vi "Main.vi"() -> ()   [LabVIEW 2018, in "TestStand_Control.lvlib"]
doc: "This template is based off of the Queued Message Handler design pattern and the Queued Message Handler project template that ships with LabVIEW.\n\nThe main difference is that the queue is private to this module and communication between modules is performed via Broadcast and Request events.\n\nRequest events are wrapped in public API methods and are handled in the Event Handling Loop (EHL) of this VI. Any module can register for Broadcast events sent by this module. The EHL generates messages based on user interface actions.\n\nThe Message Handling Loop (MHL) processes messages generated by the EHL, or by other messages. The messages are string values, so new messages can be added easily to the Message Cases case structure in the MHL. Each message cluster can also provide an optional value for Message Data, which is a variant that can be converted to whatever message-specific data is required.\n_____\nBased on Delacor QMH Project Template 4.2.1.64."
uses:
  TestStand_Control.lvlib
  <vilib>/Delacor/Delacor QMH/Libraries/Module Admin_class/Delacor_lib_QMH_Module Admin.lvclass
  Module Data--cluster.ctl
  Module_Controls/TestStand UI Data.ctl
  Stop Argument--cluster.ctl
  <vilib>/Delacor/Delacor QMH/Libraries/Message Queue_class/Delacor_lib_QMH_Message Queue.lvclass/Delacor_lib_QMH_Message Queue.ctl
  <vilib>/Delacor/Delacor QMH/Libraries/Module Admin_class/Delacor_lib_QMH_Module Admin.lvclass/Delacor_lib_QMH_Module Admin.ctl
  User_Selected_TestCase Argument--cluster.ctl
  Start_Execution Argument--cluster.ctl
  <vilib>/Utility/miscctls.llb/LVPointTypeDef.ctl
  <vilib>/Delacor/Delacor QMH/Libraries/Message Queue_class/Delacor_lib_QMH_Enqueue Message (Single).vi
  <vilib>/Delacor/Delacor QMH/Libraries/Module Admin_class/Delacor_lib_QMH_Get External Launch.vi
  <vilib>/Utility/error.llb/Error Cluster From Error Code.vi
  <vilib>/ErrorRing/Error Ring.xnode
  <vilib>/Delacor/Delacor QMH/Libraries/Message Queue_class/Delacor_lib_QMH_Message Queue.lvclass
panel:
  in  "Subpanel Ref":refnum<vi>
  in  "TestStand UI SequenceView Control":refnum<k7>(container)
  in  "Path":path
  in  "Entry Point 1 Button":refnum<k7>(container)
  in  "Start":bool
  in  "Break":refnum<k7>(container)
  in  "Terminate":refnum<k7>(container)
  in  "Test_Case":string
  in  "SequenceView Control":refnum<k7>(container)
  in  "ExecutionView Manager":refnum<k7>(container)
  in  "SequenceFileView Manager":refnum<k7>(container)
  in  "Application Manager":refnum<k7>(container)
  out "error out":errorcluster
  in  "Module Admin":refnum<class "Delacor_lib_QMH_Module Admin.lvclass">
  out "Status":string
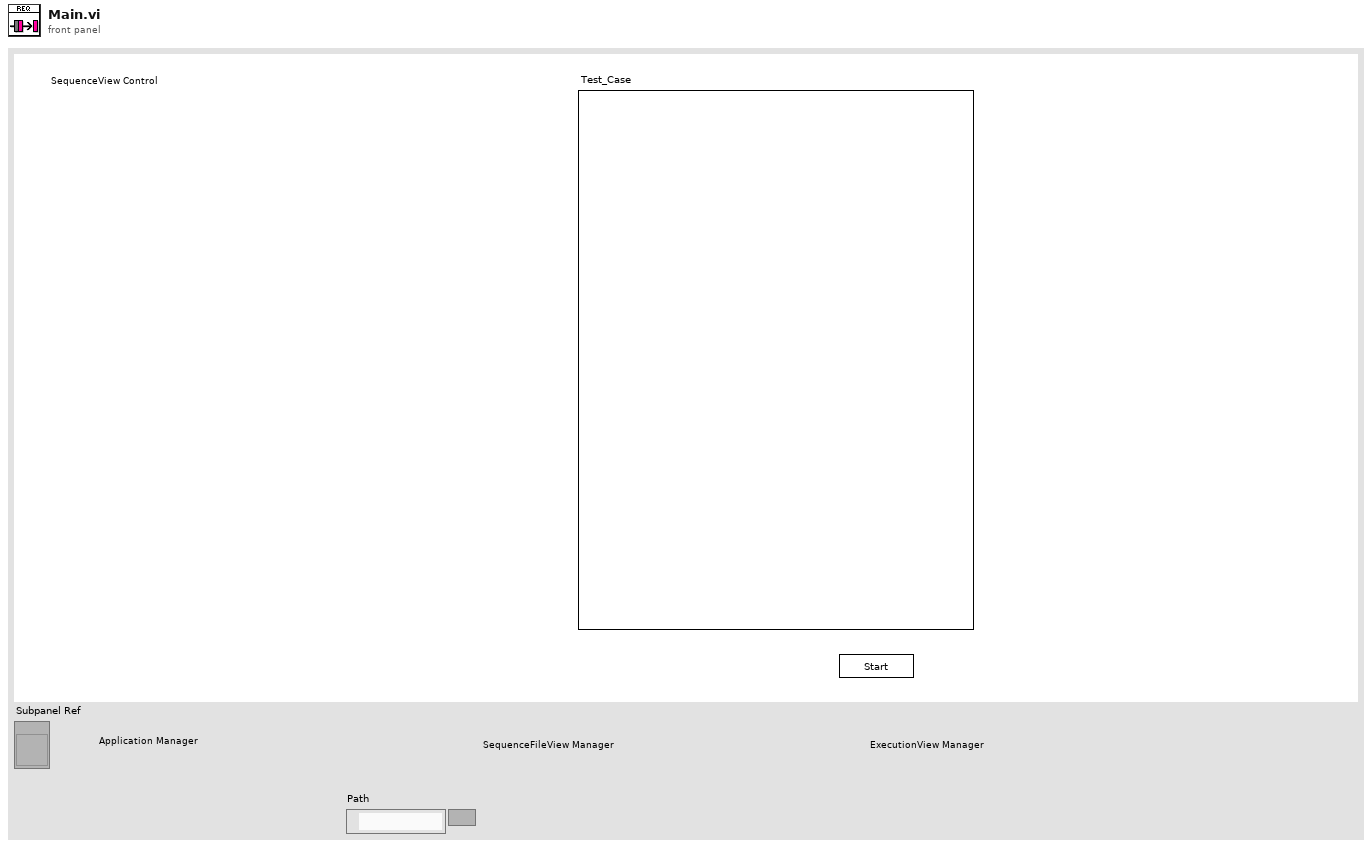
[diagram p1: front panel]
types:
  T1 = typedef "TestStand_Control.lvlib/Module Data--cluster.ctl" = cluster{"Status":string, "TestStand UI Data":T2, "Test_ID":string[], "Test_ID User":string[], "Test_Case":string[], "Subpanel Ref":refnum<vi>, "Working_Directory":path}
  T2 = typedef "TestStand_Control.lvlib/TestStand UI Data.ctl" = cluster{"Other References":cluster{"Event Callback":refnum<k27>, "Quit Application Event":refnum<user-event>, "Event Reg Refnum":refnum<event-registration>, "Top level VI":refnum<vi>, "TestStand Engine":refnum<k7>}, "Manager Controls":cluster{"Application Manager":refnum<k7>, "SequenceFileView Manager":refnum<k7>, "ExecutionView Manager":refnum<k7>}, "Visible Controls":cluster{"Terminate/Restart Button":refnum<k7>, "Break/Resume Button":refnum<k7>, "Close Executions Button":refnum<k7>, "Report Viewer":refnum<k7>, "Execution View":refnum<k7>, "Executions ComboBox":refnum<k7>, "Run Selected Sequence Button":refnum<k7>, "Entry Point 2 Button":refnum<k7>, "Entry Point 1 Button":refnum<k7>, "Close Sequence File Button":refnum<k7>, "Open Sequence File Button":refnum<k7>, "Sequences ComboBox":refnum<k7>, "Sequence Files ComboBox":refnum<k7>, "Terminate All Button":refnum<k7>, "Exit Button":refnum<k7>, "Login/Logout Button":refnum<k7>}}
  T3 = typedef "TestStand_Control.lvlib/Request Events--cluster.ctl" = cluster{"Stop Module":refnum<user-event>, "Show Panel":refnum<user-event>, "Hide Panel":refnum<user-event>, "Get Module Execution Status":refnum<user-event>, "Show Diagram":refnum<user-event>, "User_Selected_TestCase":refnum<user-event>, "Start_Execution":refnum<user-event>}
  T4 = enum32{"invalid lock state", "Not Locked", "Locked (No Password)", "Password-protected"}
  T5 = typedef "TestStand_Control.lvlib/Stop Argument--cluster.ctl" = cluster{"Origin":string, "Exit via Stop Module Req?":bool, "Wait for Module to stop?":bool}
  T6 = enum8{"Enabled", "Disabled", "Disabled and Grayed Out"}
  T7 = typedef "TestStand_Control.lvlib/User_Selected_TestCase Argument--cluster.ctl" = cluster{"Test_Case_ID":string[]}
  T8 = typedef "TestStand_Control.lvlib/Start_Execution Argument--cluster.ctl" = cluster{"Start":bool}
  T9 = typedef "LVPointTypeDef.ctl" = cluster{"Horizontal":i16, "Vertical":i16}
  T10 = enum32{"Invalid", "Standard", "Closed", "Hidden", "Minimized", "Maximized"}
  T11 = cluster{"test_id":string, "status":string, "report":string, "last":bool}
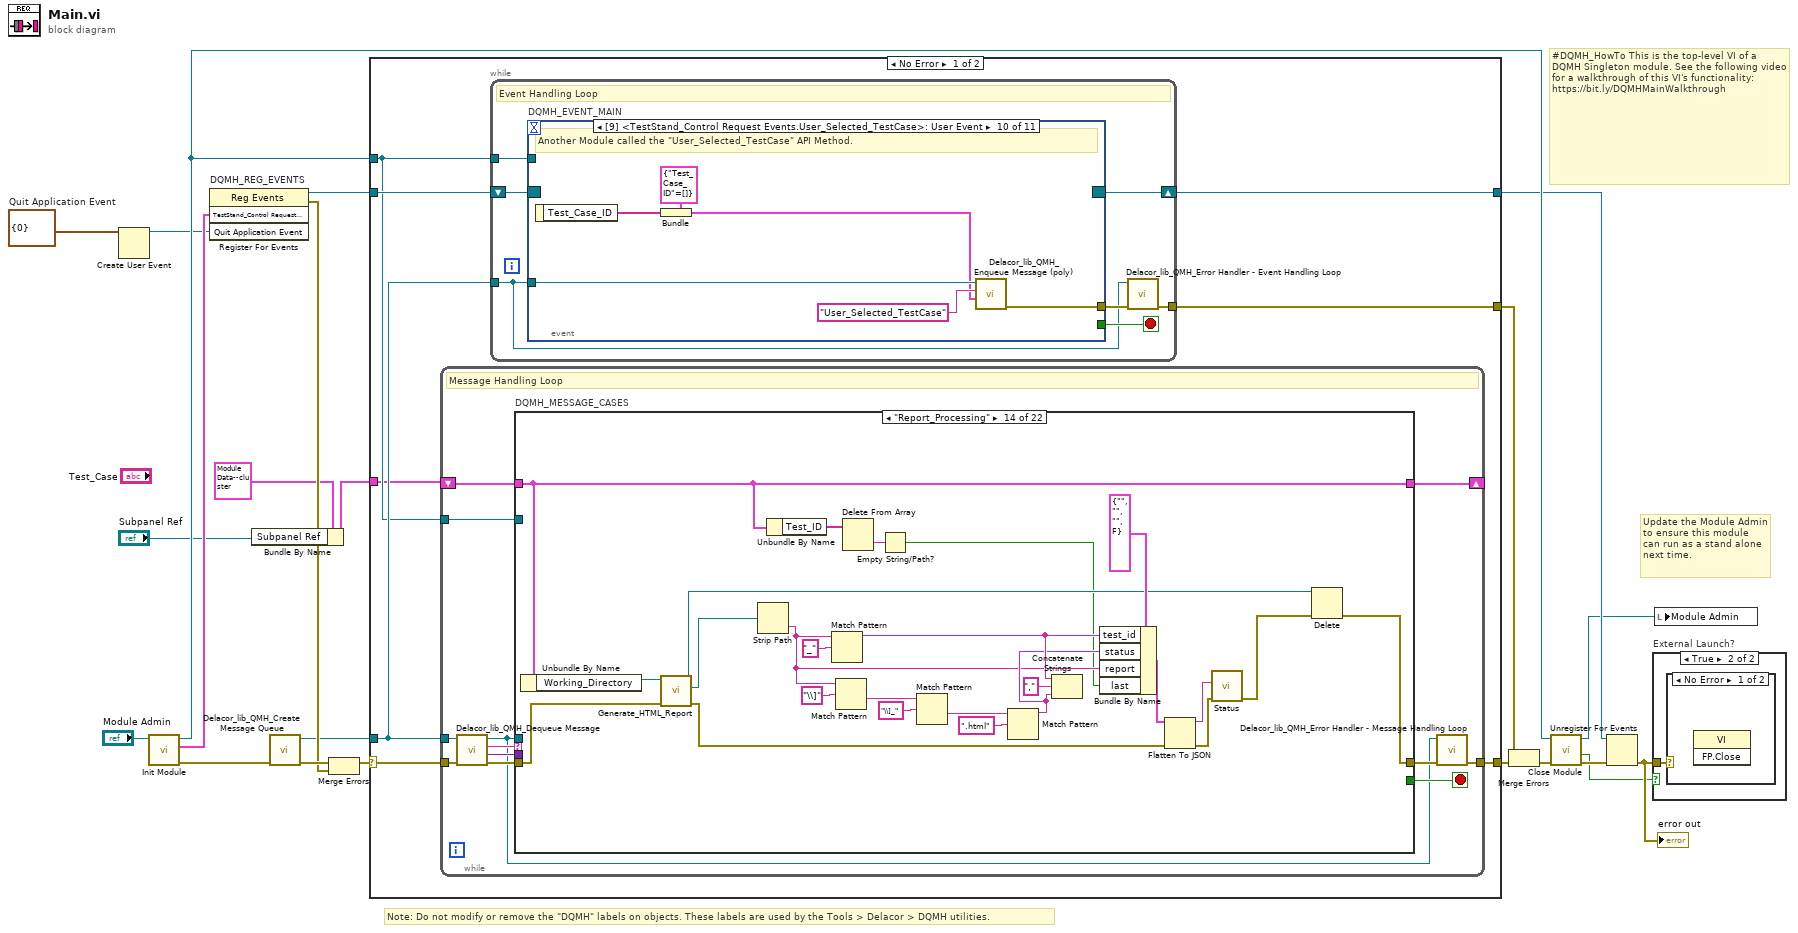
[diagram p0: block diagram]
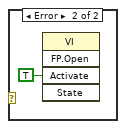
[diagram p3: hidden frame]
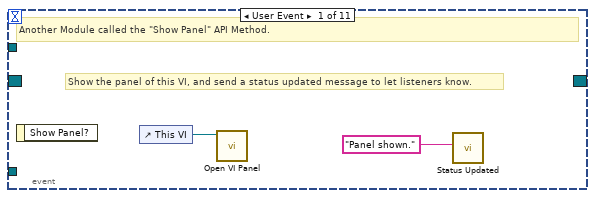
[diagram p4: hidden frame]
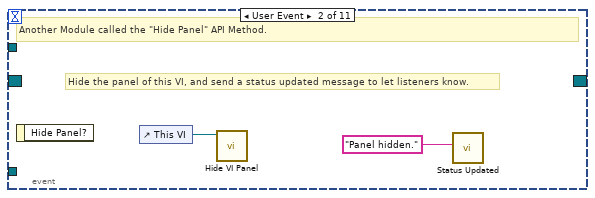
[diagram p5: hidden frame]
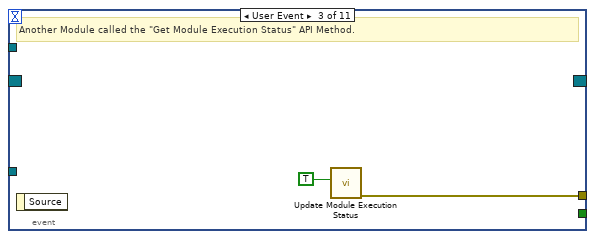
[diagram p6: hidden frame]
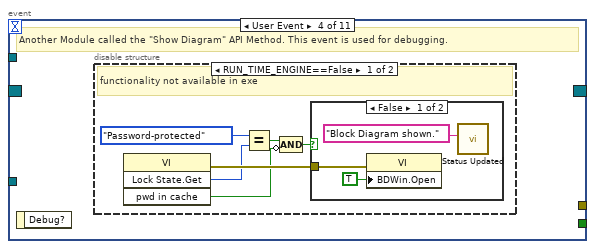
[diagram p7: hidden frame]
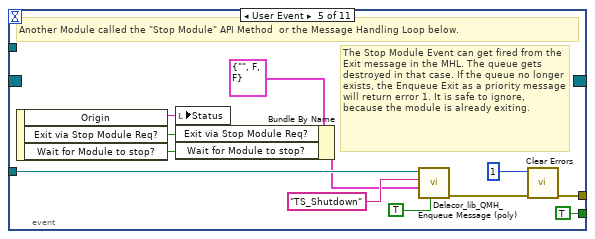
[diagram p10: hidden frame]
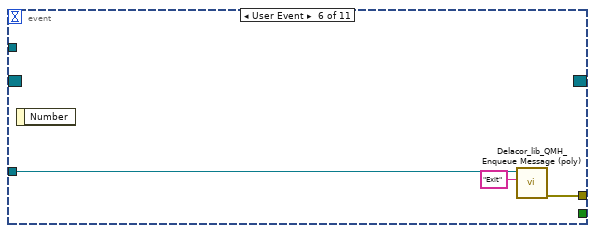
[diagram p11: hidden frame]
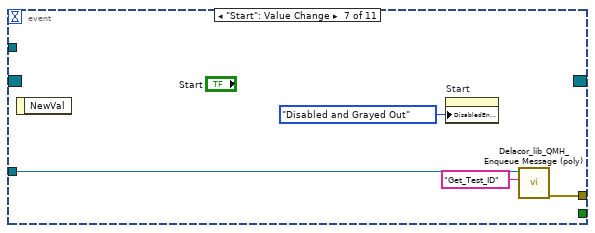
[diagram p12: hidden frame]
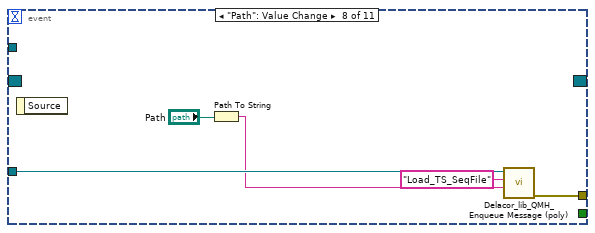
[diagram p13: hidden frame]
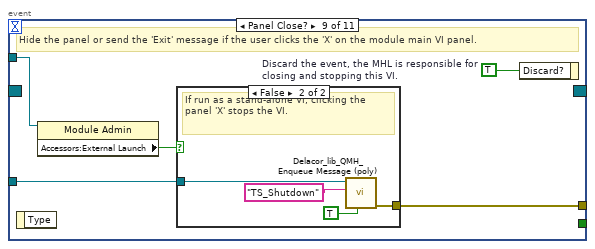
[diagram p14: hidden frame]
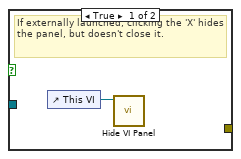
[diagram p15: hidden frame]
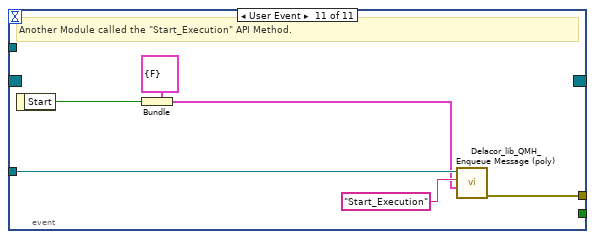
[diagram p16: hidden frame]
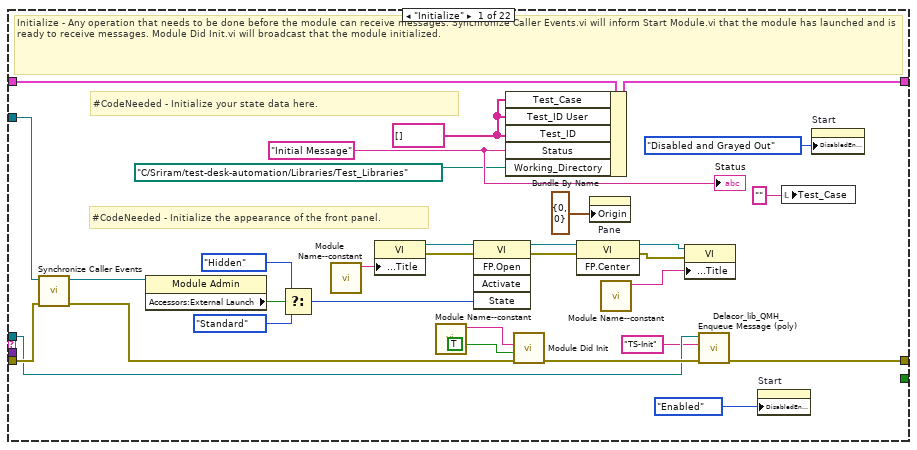
[diagram p17: hidden frame]
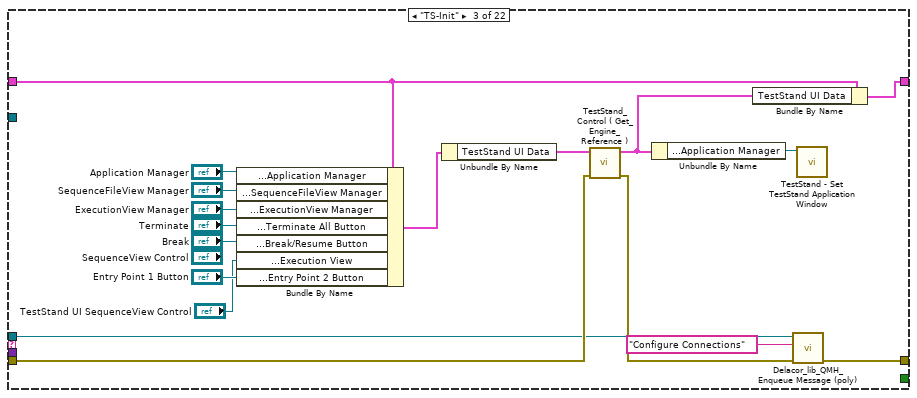
[diagram p19: hidden frame]
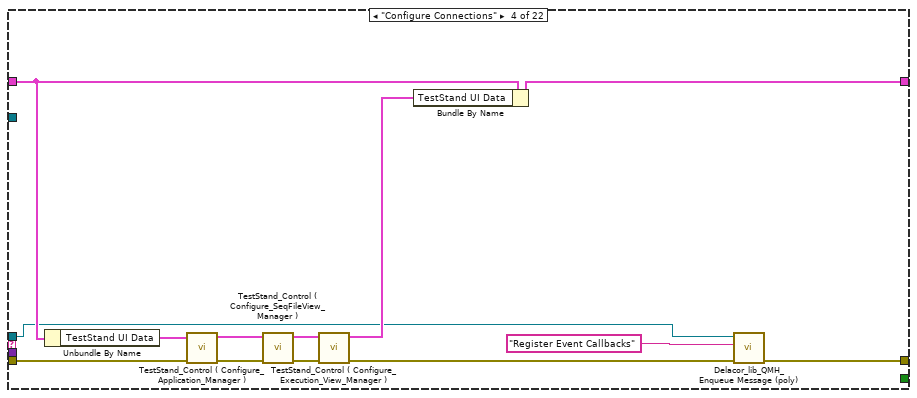
[diagram p20: hidden frame]
diagram:
  w5 = cluster{"Number":i32} {"Number"=0}  # Quit Application Event
  # "#DQMH_HowTo This is the top-level VI of a DQMH Singleton module. See the following video for a walkthrough of this VI's functionality: https://bit.ly/DQMHMainWalkthrough"
  # "Note: Do not modify or remove the \"DQMH\" labels on objects. These labels are used by the Tools > Delacor > DQMH utilities."
  # "Update the Module Admin to ensure this module can run as a stand alone next time."
  n1 = Create User Event(user event datatype=w5) -> (user event=w4:refnum<user-event>)  [unwired: 1 in, 1 out]
  n2 = call "Init Module.vi"("Singleton Module Admin in"="Module Admin") -> ("error out"=w21:errorcluster, "TestStand_Control Request Events"=w10:T3, "Singleton Module Admin out"=w13:refnum<class "Delacor_lib_QMH_Module Admin.lvclass">)  [unwired: 8 in]
  n3 = register-events "DQMH_REG_EVENTS"(w10, w4) -> (reference out=w11:refnum<event-registration>, error out=w14:errorcluster)  [unwired: 2 in]
  n4 = Bundle By Name(cluster=T1 {"Status"="", "TestStand UI Data"={"Other References"={"Event Callback"=refnum, "Quit Application Event"=refnum, "Event Reg Refnum"=refnum, "Top level VI"=refnum, "TestStand Engine"=refnum}, "Manager Controls"={"Application Manager"=refnum, "SequenceFileView Manager"=refnum, "ExecutionView Manager"=refnum}, "Visible Controls"={"Terminate/Restart Button"=refnum, "Break/Resume Button"=refnum, "Close Executions Button"=refnum, "Report Viewer"=refnum, "Execution View"=refnum, "Executions ComboBox"=refnum, "Run Selected Sequence Button"=refnum, "Entry Point 2 Button"=refnum, "Entry Point 1 Button"=refnum, "Close Sequence File Button"=refnum, "Open Sequence File Button"=refnum, "Sequences ComboBox"=refnum, "Sequence Files ComboBox"=refnum, "Terminate All Button"=refnum, "Exit Button"=refnum, "Login/Logout Button"=refnum}}, "Test_ID"=[], "Test_ID User"=[], "Test_Case"=[], "Subpanel Ref"=refnum, "Working_Directory"=path ""} ("Data Cluster"), "Subpanel Ref"="Subpanel Ref") -> (w2:T1)
  n5 = call <vilib>:"Delacor_lib_QMH_Create Message Queue.vi"("error in (no error)"=w21) -> ("error out"=w16:errorcluster, "Message Queue"=w9:refnum<class "Delacor_lib_QMH_Message Queue.lvclass">)  [unwired: 9 in]
  n6 = Merge Errors(w16, w14) -> (w15:errorcluster)
  n7 = case shown="No Error" w15 {
    selector: w15 -> [w28 w423]
    tunnel: [w30 w423] -> w22
    tunnel: [w27 w420] -> w12
    tunnel: w11 -> [w26 w420]
    tunnel: w9 -> [w25 _]
    tunnel: [w29 _] -> w19
    tunnel: w13 -> [w24 w416]
    tunnel: w2 -> [w23 _]
    frame No Error {
      n8 = while {
        tunnel: w25 -> [w101]
        shift-right: [w105] -> _
        shift-left: w23 -> [w106]
        tunnel: w28 -> [w109]
        tunnel: [w107] -> w30
        tunnel: w24 -> [w99]
        stop <- w104 stop-if-true
        # "Message Handling Loop"
        n9 = call-dynamic "Delacor_lib_QMH_Dequeue Message.vi"("error in (no error)"=w109, "Message Queue in"=w101) -> ("error out"=w108:errorcluster, "Message Data"=w102:variant, "Message"=w103:string, "Message Queue out"=w100:refnum<class "Delacor_lib_QMH_Message Queue.lvclass">)  [unwired: 6 in]
        n10 = case "DQMH_MESSAGE_CASES" shown="\"Report_Processing\"" w103 {
          selector: w103 -> [_ _ _ _ _ _ _ _ _ _ _ _ _ _ _ _ _ _ _ _ _ w403]
          tunnel: w100 -> [w121 _ w150 w162 w179 _ w202 _ _ _ _ w262 w272 _ w307 w322 w341 _ _ w369 w396 _]
          tunnel: w108 -> [w139 w143 w153 w174 w180 w190 w204 w222 w246 w249 w258 w264 w273 w301 w305 w340 w349 w364 w366 w376 w401 w405]
          tunnel: [w122 w143 w152 w164 w181 w190 w203 w223 w239 w247 w257 w263 w266 w300 w310 w318 w343 w363 w366 w372 w399 w406] -> w110
          tunnel: w106 -> [w129 w142 w147 w172 w189 w193 w205 w227 w238 w250 w252 w259 w276 w280 w313 w334 w348 w362 w365 w371 w384 w404]
          tunnel: [w112 w142 w146 w167 w188 w193 w200 w226 w238 w250 w252 w259 w276 w280 w313 w330 w348 w362 w365 w371 w384 w404] -> w105
          tunnel: [_ _ _ _ _ _ _ _ _ _ _ _ _ _ _ _ _ _ _ _ w395 _] -> w104
          tunnel: w102 -> [_ _ _ _ _ _ _ _ w243 _ w255 _ _ _ _ w339 w347 _ _ w370 w394 _]
          tunnel: w99 -> [w130 _ _ _ _ _ _ _ _ _ _ _ _ _ _ _ _ _ _ w368 w389 _]
          frame "Initialize" {
            w116 = string[] [] ("Test_ID")
            w124 = "Initial Message" ("Initial Message")
            # "#CodeNeeded - Initialize the appearance of the front panel."
            # "#CodeNeeded - Initialize your state data here."
            # "Initialize - Any operation that needs to be done before the module can receive messages. Synchronize Caller Events.vi will inform Start Module.vi that the module has launched and is ready to receive messages. Module Did Init.vi will broadcast that the module initialized."
            n11 = call "Synchronize Caller Events.vi"("error in (no error)"=w139, "Singleton Module Admin in"=w130) -> ("error out"=w138:errorcluster, "Singleton Module Admin out"=w126:refnum<class "Delacor_lib_QMH_Module Admin.lvclass">)  [unwired: 8 in]
            n12 = property class="Module Admin"(reference=w126) -> ("Accessors:External Launch"=w134:bool)  [unwired: 1 in, 2 out]
            n13 = Select(t=T10."Hidden" ("State"), s=w134, f=T10."Standard" ("State")) -> (s? t:f=w131:T10)
            n14 = call "Module Name--constant.vi"() -> ("Module Name"=w137:string)  [unwired: 11 in]
            n15 = property class="VI"("Front Panel.Title"=w137) -> (reference out=w136:refnum<vi>, error out=w141:errorcluster)  [unwired: 2 in]
            n16 = call "Module Name--constant.vi"() -> ("Module Name"=w127:string)  [unwired: 11 in]
            n17 = invoke class="VI" method="FP.Open"(reference=w136, error in=w141, "State"=w131) -> (reference out=w135:refnum<vi>, error out=w140:errorcluster)  [unwired: 2 in, 3 out]
            n18 = Bundle By Name(cluster=w129, "Test_Case"=w116, "Test_ID User"=w116, "Test_ID"=w116, "Status"=w124, "Working_Directory"=path "C:/Sriram/test-desk-automation/Libraries/Test_Libraries") -> (w112:T1)
            n19 = call "Module Did Init.vi"("error in (no error)"=w138, "Initialized?"=TRUE, "Origin"=w127) -> ("error out"=w123:errorcluster)  [unwired: 8 in]
            n20 = invoke class="VI" method="FP.Center"(reference=w135, error in=w140) -> (reference out=w114:refnum<vi>, error out=w115:errorcluster)  [unwired: 1 in, 1 out]
            n21 = property on="Pane" class="Pane"("Origin"=T9 {"Horizontal"=0, "Vertical"=0}) -> ()  [unwired: 2 in, 2 out]
            n22 = call "Module Name--constant.vi"() -> ("Module Name"=w113:string)  [unwired: 11 in]
            n23 = property class="VI"(reference=w114, error in=w115, "Front Panel.Title"=w113) -> ()  [unwired: 2 out]
            n24 = call-poly <vilib>:"Delacor_lib_QMH_Enqueue Message (poly).vi"("error in (no error)"=w123, "Message"="TS-Init", "Message Queue in"=w121) -> ("error out"=w122:errorcluster)  [unwired: 7 in, 1 out]
            n25 = property on="Start" class="Bool"("DisabledEnum"=T6."Enabled" ("Disabled")) -> ()  [unwired: 2 in, 2 out]
            n26 = local write "Test_Case"("" ("Test_Case")) -> ()
            n27 = property on="Start" class="Bool"("DisabledEnum"=T6."Disabled and Grayed Out" ("Disabled")) -> ()  [unwired: 2 in, 2 out]
            "Status" <- w124
          }
          frame "--- Module Specific ---" {
            # "Separator -- The following cases handle messages specific to this Module."
          }
          frame "TS-Init" {
            n28 = Bundle By Name(cluster=w147, "TestStand UI Data.Manager Controls.Application Manager"="Application Manager", "TestStand UI Data.Manager Controls.SequenceFileView Manager"="SequenceFileView Manager", "TestStand UI Data.Manager Controls.ExecutionView Manager"="ExecutionView Manager", "TestStand UI Data.Visible Controls.Terminate All Button"="Terminate", "TestStand UI Data.Visible Controls.Break/Resume Button"="Break", "TestStand UI Data.Visible Controls.Execution View"="TestStand UI SequenceView Control", "TestStand UI Data.Visible Controls.Entry Point 2 Button"="Entry Point 1 Button") -> (w155:T1)
            n29 = Unbundle By Name(w155) -> ("TestStand UI Data"=w154:T2)
            n30 = call "TestStand_Control ( Get_Engine_Reference ).vi"("error IO"=w153, "TestStand UI Data"=w154) -> ("error IO 2"=w151:errorcluster, "TestStand UI Data 2"=w145:T2)  [unwired: 8 in]
            n31 = Unbundle By Name(w145) -> ("Manager Controls.Application Manager"=w161:refnum<k7>)
            n32 = Bundle By Name(cluster=w147, "TestStand UI Data"=w145) -> (w146:T1)
            n33 = call-poly <vilib>:"Delacor_lib_QMH_Enqueue Message (poly).vi"("error in (no error)"=w151, "Message"="Configure Connections", "Message Queue in"=w150) -> ("error out"=w152:errorcluster)  [unwired: 7 in, 1 out]
            n34 = call <vilib>:"TestStand - Set TestStand Application Window.vi"("Application Manager"=w161) -> ()  [unwired: 2 in, 9 out]
          }
          frame "Configure Connections" {
            n35 = Unbundle By Name(w172) -> ("TestStand UI Data"=w171:T2)
            n36 = call "TestStand_Control ( Configure_Application_Manager ).vi"("error IO"=w174, "TestStand UI Data"=w171) -> ("error IO 2"=w173:errorcluster, "TestStand UI Data 2"=w169:T2)  [unwired: 8 in]
            n37 = call "TestStand_Control ( Configure_SeqFileView_Manager ).vi"("error IO"=w173, "TestStand UI Data"=w169) -> ("error IO"=w170:errorcluster, "TestStand UI Data 2"=w168:T2)  [unwired: 8 in]
            n38 = call "TestStand_Control ( Configure_Execution_View_Manager ).vi"("error IO 2"=w170, "TestStand UI Data"=w168) -> ("error IO"=w163:errorcluster, "TestStand UI Data 2"=w166:T2)  [unwired: 8 in]
            n39 = Bundle By Name(cluster=w172, "TestStand UI Data"=w166) -> (w167:T1)
            n40 = call-poly <vilib>:"Delacor_lib_QMH_Enqueue Message (poly).vi"("error in (no error)"=w163, "Message"="Register Event Callbacks", "Message Queue in"=w162) -> ("error out"=w164:errorcluster)  [unwired: 7 in, 1 out]
          }
          frame "Register Event Callbacks" {
            n41 = vi-ref "TestStand_Control ( Display_Sequence_Callback ).vi"() -> ("vi reference"=w185:refnum<vi>)
            n42 = vi-ref "TestStand_Control ( End_Execution ).vi"() -> ("vi reference"=w182:refnum<vi>)
            n43 = vi-ref "TestStand_Control ( Execution_View_Callback ).vi"() -> ("vi reference"=w184:refnum<vi>)
            n44 = vi-ref "TestStand_Control ( Start_Execution ).vi"() -> ("vi reference"=w183:refnum<vi>)
            n45 = vi-ref "TestStand_Control ( Exit_Callback ).vi"() -> ("vi reference"=w186:refnum<vi>)
            n46 = vi-ref "TestStand_Control ( Display_Execution ).vi"() -> ("vi reference"=w175:refnum<vi>)
            n47 = Unbundle By Name(w189) -> ("TestStand UI Data.Manager Controls.Application Manager"=w177:refnum<k7>, "TestStand UI Data"=w176:T2)
            n48 = node(w177, w185, w176, w177, w186, w176, w177, w184, w176, w177, w183, w179, w177, w182, w179, w177, w175, w176) -> (w187:refnum<k27>)  [unwired: 2 in, 1 out]
            n49 = call-poly <vilib>:"Delacor_lib_QMH_Enqueue Message (poly).vi"("error in (no error)"=w180, "Message"="Start Application", "Message Queue in"=w179) -> ("error out"=w181:errorcluster)  [unwired: 7 in, 1 out]
            n50 = Bundle By Name(cluster=w189, "TestStand UI Data.Other References.Event Callback"=w187) -> (w188:T1)
          }
          frame "Start Application" {
            n51 = Unbundle By Name(w193) -> ("TestStand UI Data.Manager Controls.Application Manager"=w194:refnum<k7>)
            n52 = invoke class="IApplicationMgr" method="Start"(reference=w194, error in=w190) -> (error out=w191:errorcluster)  [unwired: 1 in, 2 out]
            n53 = property on="Start" class="Bool"(error in=w191, "DisabledEnum"=T6."Enabled" ("Disabled")) -> ()  [unwired: 1 in, 2 out]
          }
          frame "Get_Test_ID" {
            n54 = Unbundle By Name(w205) -> ("Test_ID"=w201:string[], "Test_Case"=w196:string[])
            n55 = Delete From Array(array=w196) -> (deleted portion=w195:string)  [unwired: 2 in, 1 out]
            n56 = Delete From Array(array=w201) -> (deleted portion=w197:string, array with subset deleted=w199:string[])  [unwired: 2 in]
            n57 = Empty String/Path?(string/path=w197) -> (empty?=w198:bool)
            n58 = local write "Test_Case"(w195) -> ()
            n59 = case shown="False" w198 {
              tunnel: w204 -> [w217 w221]
              tunnel: [w212 w220] -> w203
              tunnel: w202 -> [w216 w219]
              tunnel: w197 -> [w214 _]
              frame False {
                n60 = call-poly <vilib>:"Delacor_lib_QMH_Enqueue Message (poly).vi"("error in (no error)"=w217, "Message Data"=w214, "Message"="Load_TS_SeqFile", "Message Queue in"=w216) -> ("error out"=w209:errorcluster, "Message Queue out"=w207:refnum<class "Delacor_lib_QMH_Message Queue.lvclass">)  [unwired: 6 in]
                n61 = call-poly <vilib>:"Delacor_lib_QMH_Enqueue Message (poly).vi"("error in (no error)"=w209, "Message Data"="TS_SetSeqView" ("Message"), "Message"="Switch_View", "Message Queue in"=w207) -> ("error out"=w208:errorcluster, "Message Queue out"=w206:refnum<class "Delacor_lib_QMH_Message Queue.lvclass">)  [unwired: 6 in]
                n62 = call-poly <vilib>:"Delacor_lib_QMH_Enqueue Message (poly).vi"("error in (no error)"=w208, "Message"="Trigger", "Message Queue in"=w206) -> ("error out"=w212:errorcluster)  [unwired: 7 in, 1 out]
              }
              frame True {
                n63 = call-poly <vilib>:"Delacor_lib_QMH_Enqueue Message (poly).vi"("error in (no error)"=w221, "Message"="Completed", "Message Queue in"=w219) -> ("error out"=w220:errorcluster)  [unwired: 7 in, 1 out]
              }
            }
            n64 = Bundle By Name(cluster=w205, "Test_ID"=w199) -> (w200:T1)
          }
          frame "Completed" {
            n65 = disable-structure shown="Disabled" {
              disable-tunnel: [w232 _] -> w223
              disable-tunnel: w222 -> [w231 _]
              frame Disabled {
                n66 = Flatten To JSON(anything=cluster{"status":string} {"status"="finished"}, error in (no error)=w231) -> (JSON string=w228:string, 11:w229:errorcluster)  [unwired: 1 in]
                n67 = call "Status.vi"("error in (no error)"=w229, "TS_Status"=w228) -> ("error out"=w232:errorcluster)  [unwired: 9 in]
              }
              frame Enabled {
              }
            }
            n68 = property on="Start" class="Bool"("DisabledEnum"=T6."Enabled" ("Disabled")) -> ()  [unwired: 2 in, 2 out]
            n69 = Bundle By Name(cluster=w227, "Test_ID"=string[] []) -> (w226:T1)
          }
          frame "Load_TS_SeqFile" {
            n70 = Variant To Data(error in=w246, type="", Variant=w243) -> (data=w241:string, error out=w244:errorcluster)
            n71 = Unbundle By Name(w238) -> ("Working_Directory"=w236:path)
            n72 = Concatenate Strings("TestBuilds\\" ("string"), w241, ".seq" ("string")) -> (w235:string)
            n73 = Build Path(base path=w236, name or relative path=w235) -> (appended path=w234:path)
            n74 = Unbundle By Name(w238) -> ("TestStand UI Data"=w245:T2)
            n75 = Path To String(path=w234) -> (string=w233:string)
            n76 = call "TestStand_Control ( Load_Seq_File ).vi"("error in (no error)"=w244, "sequenceFilePath"=w233, "TestStand UI Data"=w245) -> ("error out"=w239:errorcluster)  [unwired: 8 in]
          }
          frame "Trigger" {
            n77 = Unbundle By Name(w250) -> ("TestStand UI Data.Visible Controls.Entry Point 2 Button"=w248:refnum<k7>)
            n78 = invoke class="IButton" method="DoClick"(reference=w248, error in=w249) -> (error out=w247:errorcluster)  [unwired: 1 in, 2 out]
          }
          frame "Switch_View" {
            n79 = Variant To Data(error in=w258, type="", Variant=w255) -> (data=w253:string, error out=w256:errorcluster)
            n80 = Unbundle By Name(w252) -> ("TestStand UI Data"=w251:T2)
            n81 = call "TestStand_Control ( Switch_View ).vi"("error in"=w256, "View"=w253, "TestStand UI Data"=w251) -> ("error out"=w257:errorcluster)  [unwired: 8 in]
          }
          frame "TS_Execution_Start" {
            n82 = call-poly <vilib>:"Delacor_lib_QMH_Enqueue Message (poly).vi"("error in (no error)"=w264, "Message Data"="TS_SetExecView" ("Message"), "Message"="Switch_View", "Message Queue in"=w262) -> ("error out"=w263:errorcluster)  [unwired: 6 in, 1 out]
          }
          frame "TS_Execution_Stop" {
            n83 = call-poly <vilib>:"Delacor_lib_QMH_Enqueue Message (poly).vi"("error in (no error)"=w273, "Message Data"="TS_SetSeqView" ("Message"), "Message"="Switch_View", "Message Queue in"=w272) -> ("error out"=w271:errorcluster, "Message Queue out"=w270:refnum<class "Delacor_lib_QMH_Message Queue.lvclass">)  [unwired: 6 in]
            n84 = call-poly <vilib>:"Delacor_lib_QMH_Enqueue Message (poly).vi"("error in (no error)"=w271, "Message"="Report_Processing", "Message Queue in"=w270) -> ("error out"=w267:errorcluster, "Message Queue out"=w265:refnum<class "Delacor_lib_QMH_Message Queue.lvclass">)  [unwired: 7 in]
            n85 = call-poly <vilib>:"Delacor_lib_QMH_Enqueue Message (poly).vi"("error in (no error)"=w267, "Message"="Get_Test_ID", "Message Queue in"=w265) -> ("error out"=w266:errorcluster)  [unwired: 7 in, 1 out]
          }
          frame "Report_Processing" {
            n86 = Unbundle By Name(w280) -> ("Working_Directory"=w282:path)
            n87 = call "Generate_HTML_Report.vi"("error in (no error)"=w301, "Working_Dir"=w282) -> ("error IO"=w285:errorcluster, "HTML_Path"=w299:path, "XML_Path"=w281:path)  [unwired: 7 in]
            n88 = Strip Path(path=w299) -> (name=w287:string)  [unwired: 1 out]
            n89 = Unbundle By Name(w280) -> ("Test_ID"=w279:string[])
            n90 = Match Pattern(string=w287, regular expression="_") -> (before substring=w289:string)  [unwired: 1 in, 3 out]
            n91 = Match Pattern(string=w287, regular expression="\\]" ("string")) -> (after substring=w292:string)  [unwired: 1 in, 3 out]
            n92 = Delete From Array(array=w279) -> (deleted portion=w278:string)  [unwired: 2 in, 1 out]
            n93 = Empty String/Path?(string/path=w278) -> (empty?=w277:bool)
            n94 = Match Pattern(string=w292, regular expression="\\]_" ("string")) -> (after substring=w291:string)  [unwired: 1 in, 3 out]
            n95 = Match Pattern(string=w291, regular expression=".html") -> (before substring=w288:string)  [unwired: 1 in, 3 out]
            n96 = Concatenate Strings(w289, "," ("string"), w288) -> ()  [unwired: 1 out]
            n97 = Bundle By Name(cluster=T11 {"test_id"="", "status"="", "report"="", "last"=FALSE} ("Cluster"), "test_id"=w289, "status"=w288, "report"=w287, "last"=w277) -> (w286:T11)
            n98 = Flatten To JSON(anything=w286, error in (no error)=w285) -> (JSON string=w284:string, 11:w283:errorcluster)  [unwired: 1 in]
            n99 = call "Status.vi"("error in (no error)"=w283, "TS_Status"=w284) -> ("error out"=w298:errorcluster)  [unwired: 9 in]
            n100 = Delete(path (use dialog)=w281, error in=w298) -> (error out=w300:errorcluster)  [unwired: 3 in, 2 out]
          }
          frame "TS_Shutdown" {
            n101 = Unbundle By Name(w313) -> ("TestStand UI Data.Manager Controls.Application Manager"=w312:refnum<k7>, "TestStand UI Data"=w304:T2)
            n102 = call "TestStand_Control ( Close_Seq ).vi"("error in (no error)"=w305, "TestStand UI Data"=w304) -> ("error out"=w303:errorcluster)  [unwired: 9 in]
            n103 = invoke class="IApplicationMgr" method="Shutdown"(reference=w312, error in=w303) -> (error out=w302:errorcluster, "Shutdown"=w311:bool)  [unwired: 1 in, 1 out]
            n104 = Select(t="Exit", s=w311, f="TS_Shutdown") -> (s? t:f=w308:string)
            n105 = call-poly <vilib>:"Delacor_lib_QMH_Enqueue Message (poly).vi"("error in (no error)"=w302, "Message"=w308, "Message Queue in"=w307) -> ("error out"=w310:errorcluster)  [unwired: 7 in, 1 out]
          }
          frame "User_Selected_TestCase" {
            # "User Selects Testcase"
            n106 = Variant To Data(error in=w340, type=T7 {"Test_Case_ID"=[]} ("User_Selected_TestCase Argument"), Variant=w339) -> (data=w337:T7, error out=w336:errorcluster)
            n107 = Unbundle By Name(w337) -> ("Test_Case_ID"=w335:string[])
            n108 = Unbundle By Name(w334) -> ("Test_ID"=w332:string[], "Test_Case"=w325:string[], "Working_Directory"=w314:path)
            n109 = Index Array(array=w335) -> (element #1=w315:string, element #2=w316:string)  [unwired: 3 in, 1 out]
            n110 = local write "Test_Case"(w315) -> ()
            n111 = Search 1D Array(1D array=w332, element=w316) -> (index of element=w333:i32)  [unwired: 1 in]
            n112 = Greater Or Equal To 0?(x=w333) -> (x >= 0?=w326:bool)
            n113 = call "TestStand_Builder ( Test-Build ).vi"("error out"=w336, "Working_Dir"=w314, "Test_ID"=w316, "Test_Case"=w315) -> ("error out 2"=w323:errorcluster)  [unwired: 7 in]
            n114 = Build Array (concatenate)(w332, w316) -> (w331:string[])
            n115 = Build Array (concatenate)(w325, w315) -> (w327:string[])
            n116 = Select(t=w332, s=w326, f=w331) -> (s? t:f=w329:string[])
            n117 = Select(t=w325, s=w326, f=w327) -> (s? t:f=w328:string[])
            n118 = call-poly <vilib>:"Delacor_lib_QMH_Enqueue Message (poly).vi"("error in (no error)"=w323, "Message Data"=w316, "Message"="Load_TS_SeqFile", "Message Queue in"=w322) -> ("error out"=w319:errorcluster, "Message Queue out"=w317:refnum<class "Delacor_lib_QMH_Message Queue.lvclass">)  [unwired: 6 in]
            n119 = Bundle By Name(cluster=w334, "Test_ID"=w329, "Test_ID User"=w329, "Test_Case"=w328) -> (w330:T1)
            n120 = call-poly <vilib>:"Delacor_lib_QMH_Enqueue Message (poly).vi"("error in (no error)"=w319, "Message Data"="TS_SetSeqView" ("Message"), "Message"="Switch_View", "Message Queue in"=w317) -> ("error out"=w318:errorcluster)  [unwired: 6 in, 1 out]
          }
          frame "Start_Execution" {
            # "#CodeNeeded\n1. Configure this Message Case for handling the \"Start_Execution\" message.\n2. Delete or edit this label when done."
            # "Starts TestStand Execution"
            n121 = Variant To Data(error in=w349, type=T8 {"Start"=FALSE} ("Start_Execution Argument"), Variant=w347) -> (data=w345:T8, error out=w344:errorcluster)
            n122 = Unbundle By Name(w345) -> ("Start"=w342:bool)
            n123 = case shown="True" w342 {
              tunnel: w344 -> [w350 w351]
              tunnel: [w350 w354] -> w343
              tunnel: w341 -> [_ w353]
              frame False {
              }
              frame True {
                n124 = disable-structure shown="Enabled" {
                  disable-tunnel: [w360 w361] -> w352
                  disable-tunnel: w351 -> [w357 w361]
                  frame Disabled {
                    n125 = Flatten To JSON(anything=cluster{"test_action":string} {"test_action"="test_start"}, error in (no error)=w357) -> (JSON string=w359:string, 11:w358:errorcluster)  [unwired: 1 in]
                    n126 = call "Status.vi"("error in (no error)"=w358, "TS_Status"=w359) -> ("error out"=w360:errorcluster)  [unwired: 9 in]
                  }
                  frame Enabled {
                  }
                }
                n127 = call-poly <vilib>:"Delacor_lib_QMH_Enqueue Message (poly).vi"("error in (no error)"=w352, "Message"="Get_Test_ID", "Message Queue in"=w353) -> ("error out"=w354:errorcluster)  [unwired: 7 in, 1 out]
              }
            }
          }
          frame "---Copy This Frame---" {
            # "Duplicate this frame when creating new messages.  Change this comment in the duplicated frame to describe this message."
            n128 = Merge Errors(w364) -> (w363:errorcluster)
          }
          frame "--- Exit and Error Handling---" {
            # "Separator - The following cases handle errors and exit messages."
          }
          frame "Error" {
            # "#CodeRecommended - If you ever change the name of this \"Error\" message, you'll need to update the name in the Check Loop Error.vi as well."
            # "#CodeRecommended - If the module is running in standalone mode (External Launch = FALSE), this code will pop up an error dialog and call the 'Exit' message if an error occurs. Add more fine-grained error handling here."
            # "Error - Check the error message data and respond accordingly. This message is sent by the \"Error Handler\" VIs at the end of each loop in this application."
            n129 = property class="Module Admin"(reference=w368) -> ("Accessors:External Launch"=w367:bool)  [unwired: 1 in, 2 out]
            n130 = Variant To Data(error in=w376, type=errorcluster {"status"=FALSE, "code"=0, "source"=""} ("error constant"), Variant=w370) -> (data=w377:errorcluster, error out=w374:errorcluster)
            n131 = call "Error Reported.vi"("Error"=w377) -> ()  [unwired: 10 in, 1 out]
            n132 = case shown="False" w367 {
              tunnel: [w382 _] -> w373
              tunnel: w369 -> [w380 _]
              tunnel: w377 -> [w381 _]
              frame False {
                # "If the module is running standalone, then pop up an error dialog and call the \"Exit\" message."
                n133 = call <vilib>:"Simple Error Handler.vi"("error in (no error)"=w381) -> ()  [unwired: 4 in, 5 out]
                n134 = call-poly <vilib>:"Delacor_lib_QMH_Enqueue Message (poly).vi"("Priority Message? (F)"=TRUE, "Message"="Exit", "Message Queue in"=w380) -> ("error out"=w382:errorcluster)  [unwired: 7 in, 1 out]
              }
              frame True {
                # "If the module was launched externally, calling the Error Reported broadcast VI is the only action performed by the \"Error\" message. The module's caller can then process the error appropriately."
              }
            }
            n135 = Merge Errors(w374, w373) -> (w372:errorcluster)
            n136 = local write "error out"(w372) -> ()
          }
          frame "Exit" {
            w393 = 91  # 91: not all Exit messages will have an argument
            w395 = TRUE  # Stop the VI
            # "Release the message queue reference"
            # "Exit - Exit the application."
            n137 = Variant To Data(error in=w401, type=T5 {"Origin"="", "Exit via Stop Module Req?"=FALSE, "Wait for Module to stop?"=FALSE} ("Stop Argument"), Variant=w394) -> (data=w391:T5, error out=w398:errorcluster)
            n138 = call <vilib>:"Clear Errors.vi"("error in (no error)"=w398, "specific error code to clear (0: all)"=w393) -> ("error out"=w400:errorcluster)  [unwired: 4 in, 1 out]
            n139 = call-dynamic "Delacor_lib_QMH_Release Message Queue.vi"("error in (no error)"=w400, "Message Queue"=w396) -> ("error out"=w383:errorcluster)  [unwired: 9 in]
            n140 = Unbundle By Name(w384) -> ("TestStand UI Data.Other References.TestStand Engine"=w386:refnum<k7>, "TestStand UI Data.Other References.Event Callback"=w387:refnum<k27>)  [unwired: 1 out]
            n141 = Unregister For Events(event registration refnum=w387, error in=w383) -> (error out=w388:errorcluster)
            n142 = control-ref of="This VI"() -> (w390:refnum<vi>)
            n143 = call "Handle Exit.vi"("Stop Argument"=w391, "Admin in"=w389, "VI reference"=w390) -> ("error out"=w397:errorcluster)  [unwired: 7 in, 1 out]
            n144 = Close Reference(reference=w386, error in (no error)=w388) -> (error out=w385:errorcluster)
            n145 = Merge Errors(w385, w397) -> (w399:errorcluster)
          }
          frame Default {
            # "'Default' case only runs if there is a message that isn't defined in any of the other cases.  Output a programming error."
            n146 = call "Module Name--constant.vi"() -> ("Module Name"=w402:string)  [unwired: 11 in]
            n147 = xnode "Error Ring"("parameter 0"=w403, "parameter 1"=w402) -> ("error out"=w407:errorcluster)
            n148 = Merge Errors(w405, w407) -> (w406:errorcluster)
          }
        }
        n149 = call-dynamic "Delacor_lib_QMH_Error Handler - Message Handling Loop.vi"("error in (no error)"=w110, "Message Queue in"=w100) -> ("dup error in"=w107:errorcluster)  [unwired: 8 in, 1 out]
      }
      n150 = while {
        tunnel: w25 -> [w31]
        shift-right: [w34] -> w27
        shift-left: w26 -> [w35]
        tunnel: [w36] -> w29
        tunnel: w24 -> [w32]
        stop <- w33 stop-if-true
        # "Event Handling Loop"
        n151 = event "DQMH_EVENT_MAIN" shown="[9] <TestStand_Control Request Events.User_Selected_TestCase>: User Event" {
          selector: w35 -> [_ _ _ _ _ _ _ _ _ _ _]
          dyn-events: [_ _ _ _ _ _ _ _ _ _ _] -> w34
          timeout: _ -> [_ _ _ _ _ _ _ _ _ _ _]
          tunnel: [_ _ _ _ TRUE ("Discard?") _ _ _ _ _ _] -> w33
          tunnel: w31 -> [_ _ _ _ w60 w66 w70 w75 w79 w92 w98]
          tunnel: [_ _ w43 _ w63 w67 w71 w76 w81 w87 w93] -> w37
          tunnel: w32 -> [_ _ _ _ _ _ _ _ w78 _ _]
          event User Event {
            # "Show the panel of this VI, and send a status updated message to let listeners know."
            # "Another Module called the \"Show Panel\" API Method."
            n152 = event-data() -> ()  [unwired: 1 in, 1 out]
            n153 = control-ref of="This VI"() -> (w39:refnum<vi>)
            n154 = call "Open VI Panel.vi"("VI"=w39) -> ()  [unwired: 10 in, 1 out]
            n155 = call "Status Updated.vi"("Status"="Panel shown." ("format string")) -> ()  [unwired: 10 in, 1 out]
          }
          event User Event {
            # "Hide the panel of this VI, and send a status updated message to let listeners know."
            # "Another Module called the \"Hide Panel\" API Method."
            n156 = event-data() -> ()  [unwired: 1 in, 1 out]
            n157 = control-ref of="This VI"() -> (w41:refnum<vi>)
            n158 = call "Hide VI Panel.vi"("VI"=w41) -> ()  [unwired: 10 in, 1 out]
            n159 = call "Status Updated.vi"("Status"="Panel hidden." ("format string")) -> ()  [unwired: 10 in, 1 out]
          }
          event User Event {
            # "Another Module called the \"Get Module Execution Status\" API Method."
            n160 = event-data() -> ()  [unwired: 1 in, 1 out]
            n161 = call "Update Module Execution Status.vi"("Running?"=TRUE) -> ("error out"=w43:errorcluster)  [unwired: 10 in]
          }
          event User Event {
            # "Another Module called the \"Show Diagram\" API Method. This event is used for debugging."
            n162 = event-data() -> ()  [unwired: 1 in, 1 out]
            n163 = disable-structure shown="RUN_TIME_ENGINE==False" {
              frame condition #0 (active) {
                # "functionality not available in exe"
                n164 = invoke class="VI" method="Lock State.Get"() -> (error out=w49:errorcluster, "Get Lock State"=w48:T4, "pwd in cache"=w45:bool)  [unwired: 4 in, 1 out]
                n165 = Equal?(x=T4."Password-protected", y=w48) -> (x = y?=w46:bool)
                n166 = Compound Arithmetic op=AND(w46, invert w45) -> (w44:bool)
                n167 = case shown="False" w44 {
                  tunnel: w49 -> [w52 _]
                  frame False {
                    n168 = property class="VI"(error in=w52, "BDWin.Open"=TRUE ("Block Diagram Window:Open")) -> ()  [unwired: 1 in, 2 out]
                    n169 = call "Status Updated.vi"("Status"="Block Diagram shown." ("format string")) -> ()  [unwired: 10 in, 1 out]
                  }
                  frame True {
                    # "Password-protected VI, and the password is not in the cache. Do not show the diagram."
                  }
                }
              }
              frame condition #1 {
              }
            }
          }
          event User Event {
            # "The Stop Module Event can get fired from the Exit message in the MHL. The queue gets destroyed in that case. If the queue no longer exists, the Enqueue Exit as a priority message will return error 1. It is safe to ignore, because the module is already exiting."
            # "Another Module called the \"Stop Module\" API Method  or the Message Handling Loop below."
            n170 = event-data() -> ("Origin"=w59:string, "Exit via Stop Module Req?"=w55:bool, "Wait for Module to stop?"=w54:bool)  [unwired: 1 in]
            n171 = local write "Status"(w59) -> ()
            n172 = Bundle By Name(cluster=T5 {"Origin"="", "Exit via Stop Module Req?"=FALSE, "Wait for Module to stop?"=FALSE} ("Stop Argument"), "Exit via Stop Module Req?"=w55, "Wait for Module to stop?"=w54) -> (w53:T5)
            n173 = call-poly <vilib>:"Delacor_lib_QMH_Enqueue Message (poly).vi"("Priority Message? (F)"=TRUE, "Message Data"=w53, "Message"="TS_Shutdown", "Message Queue in"=w60) -> ("error out"=w64:errorcluster)  [unwired: 6 in, 1 out]
            n174 = call <vilib>:"Clear Errors.vi"("error in (no error)"=w64, "specific error code to clear (0: all)"=1) -> ("error out"=w63:errorcluster)  [unwired: 4 in, 1 out]
          }
          event User Event {
            n175 = event-data() -> ()  [unwired: 1 in, 1 out]
            n176 = call-poly <vilib>:"Delacor_lib_QMH_Enqueue Message (poly).vi"("Message"="Exit", "Message Queue in"=w66) -> ("error out"=w67:errorcluster)  [unwired: 8 in, 1 out]
          }
          event "Start": Value Change {
            n177 = event-data() -> ()  [unwired: 1 in, 1 out]
            n178 = property on="Start" class="Bool"("DisabledEnum"=T6."Disabled and Grayed Out" ("Disabled")) -> ()  [unwired: 2 in, 2 out]
            n179 = call-poly <vilib>:"Delacor_lib_QMH_Enqueue Message (poly).vi"("Message"="Get_Test_ID", "Message Queue in"=w70) -> ("error out"=w71:errorcluster)  [unwired: 8 in, 1 out]
          }
          event "Path": Value Change {
            n180 = event-data() -> ()  [unwired: 1 in, 1 out]
            n181 = Path To String(path="Path") -> (string=w73:string)
            n182 = call-poly <vilib>:"Delacor_lib_QMH_Enqueue Message (poly).vi"("Message Data"=w73, "Message"="Load_TS_SeqFile", "Message Queue in"=w75) -> ("error out"=w76:errorcluster)  [unwired: 7 in, 1 out]
          }
          event Panel Close? {
            w80 = TRUE  # Discard the event, the MHL is responsible for closing and stopping this VI.
            # "Hide the panel or send the 'Exit' message if the user clicks the 'X' on the module main VI panel."
            n183 = event-data() -> ()  [unwired: 1 in, 1 out]
            n184 = property class="Module Admin"(reference=w78) -> ("Accessors:External Launch"=w77:bool)  [unwired: 1 in, 2 out]
            n185 = case shown="False" w77 {
              tunnel: w79 -> [_ w85]
              tunnel: [_ w86] -> w81
              frame True {
                # "If externally launched, clicking the 'X' hides the panel, but doesn't close it."
                n186 = control-ref of="This VI"() -> (w82:refnum<vi>)
                n187 = call "Hide VI Panel.vi"("VI"=w82) -> ()  [unwired: 10 in, 1 out]
              }
              frame False {
                # "If run as a stand-alone VI, clicking the panel 'X' stops the VI."
                n188 = call-poly <vilib>:"Delacor_lib_QMH_Enqueue Message (poly).vi"("Priority Message? (F)"=TRUE, "Message"="TS_Shutdown", "Message Queue in"=w85) -> ("error out"=w86:errorcluster)  [unwired: 7 in, 1 out]
              }
            }
            n189 = event-data("Discard?"=w80) -> ()  [unwired: 1 in, 1 out]
          }
          event User Event {
            # "Another Module called the \"User_Selected_TestCase\" API Method."
            n190 = event-data() -> ("Test_Case_ID"=w88:string[])  [unwired: 1 in]
            n191 = Bundle(cluster=T7 {"Test_Case_ID"=[]} ("User_Selected_TestCase Argument"), "Test_Case_ID"=w88) -> (w89:T7)
            n192 = call-poly <vilib>:"Delacor_lib_QMH_Enqueue Message (poly).vi"("Message Data"=w89, "Message"="User_Selected_TestCase", "Message Queue in"=w92) -> ("error out"=w87:errorcluster)  [unwired: 7 in, 1 out]
          }
          event User Event {
            # "Another Module called the \"Start_Execution\" API Method."
            n193 = event-data() -> ("Start"=w94:bool)  [unwired: 1 in]
            n194 = Bundle(cluster=T8 {"Start"=FALSE} ("Start_Execution Argument"), "Start"=w94) -> (w95:T8)
            n195 = call-poly <vilib>:"Delacor_lib_QMH_Enqueue Message (poly).vi"("Message Data"=w95, "Message"="Start_Execution", "Message Queue in"=w98) -> ("error out"=w93:errorcluster)  [unwired: 7 in, 1 out]
          }
        }
        n196 = call-dynamic "Delacor_lib_QMH_Error Handler - Event Handling Loop.vi"("error in (no error)"=w37, "Message Queue in"=w31) -> ("dup error in"=w36:errorcluster)  [unwired: 8 in, 1 out]
      }
    }
    frame Error {
      # "Synchronize Caller Events.vi will inform Start Module.vi that the module has launched and will let the code calling Start Module.vi register for broadcasts and would permit the caller receive the broadcast that an error occurred at launch time."
      n197 = call "Synchronize Caller Events.vi"("Singleton Module Admin in"=w416) -> ("error out"=w421:errorcluster)  [unwired: 9 in, 1 out]
      n198 = call "Module Name--constant.vi"() -> ("Module Name"=w419:string)  [unwired: 11 in]
      n199 = Format Into String(format string="An error occurred during initialization. %s is no longer running.", w419) -> (resulting string=w417:string)  [unwired: 2 in, 1 out]
      n200 = Merge Errors(w423, w421) -> (w422:errorcluster)
      n201 = call "Error Reported.vi"("Additional Information"=w417, "Error"=w422) -> ()  [unwired: 9 in, 1 out]
    }
  }
  n202 = Merge Errors(w19, w22) -> (w18:errorcluster)
  n203 = call "Close Module.vi"("error in (no error)"=w18, "Module Admin in"=w13) -> ("error out"=w20:errorcluster, "External Launch"=w6:bool, "Module Admin out"=w7:refnum<class "Delacor_lib_QMH_Module Admin.lvclass">)  [unwired: 7 in]
  n204 = Unregister For Events(event registration refnum=w12, error in=w20) -> (error out=w17:errorcluster)
  "error out" <- w17
  n205 = case "External Launch?" shown="True" w6 {
    tunnel: w17 -> [_ w424]
    frame False {
    }
    frame True {
      n206 = case shown="No Error" w424 {
        frame No Error {
          n207 = invoke class="VI" method="FP.Close"() -> ()  [unwired: 3 in, 3 out]
        }
        frame Error {
          n208 = invoke class="VI" method="FP.Open"("Activate"=TRUE ("Activate?")) -> ()  [unwired: 4 in, 5 out]
        }
      }
    }
  }
  n209 = local write "Module Admin"(w7) -> ()
